vi "Begin.vi"(8 "error in":errorcluster) -> (0 "error out":errorcluster)   [LabVIEW 2020]
doc: "Called before other user functions, this VI is expected to open initial I/O refnums, load in file data, and do all program initialization. Notice that the <B>error out</B> terminal is simply used for data flow. Wiring it to other structures or subVIs ensures that this VI runs first."
uses:
  <vilib>/Rock Robotics/WPI/DriverStation/WPI_DriverStationRobotMode2.ctl
  <vilib>/Rock Robotics/WPI/Joystick/WPI_JoystickDeviceEnum.ctl
  Robot Global Data.vi
  <vilib>/Rock Robotics/WPI/RobotDrive/WPI_RobotDriveOpen2MotorWithExistingMotors.vi
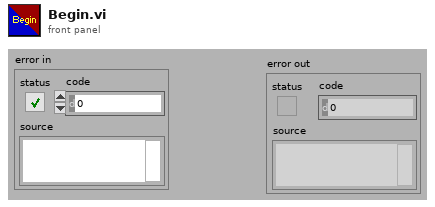
[diagram p1: front panel]
types:
  T1 = typedef "WPI_JoystickDeviceEnum.ctl" = enum16{"USB 0", "USB 1", "USB 2", "USB 3", "USB 4", "USB 5"}
  T2 = typedef "WPI_DriverStationRobotMode2.ctl" = enum16{"Autonomous Disabled", "Autonomous Enabled", "Teleop Disabled", "Teleop Enabled", "Disconnected", "Finish", "Test Disabled", "Test Enabled", "Emergency Stopped"}
  T3 = typedef "WPI_JoystickDevRef.ctl" = cluster{"Device":T1}
  T4 = typedef "WPI_MotorControlDeviceRef.ctl" = cluster{"DeviceStatus":errorcluster, "Type":T5, "PWM":cluster{"PWM Channel":T6, "DeadBand":T7}, "CAN":cluster{"Device Number":u8, "SetOutput VI Ref":variant, "GetOutput VI Ref":variant, "Enable VI Ref":variant, "Disable VI Ref":variant, "Data":variant}, "Invert":bool, "DIO PWM":cluster{"PWM \"Enable\" Channel":T6, "DIOChannel":T8, "PWM Rate":dbl}}
  T5 = typedef "WPI_MotorControlType.ctl" = enum16{"PWM", "CAN", "DIO PWM"}
  T6 = typedef "FPGA_DIOPWMChannel.ctl" = enum8{"PWM 0", "PWM 1", "PWM 2", "PWM 3", "PWM 4", "PWM 5", "PWM 6", "PWM 7", "PWM 8", "PWM 9", "PWM MXP 0", "PWM MXP 1", "PWM MXP 2", "PWM MXP 3", "PWM MXP 4", "PWM MXP 5", "PWM MXP 6", "PWM MXP 7", "PWM MXP 8", "PWM MXP 9", "Invalid"}
  T7 = typedef "WPI_PWMDeadband.ctl" = cluster{"Name":string, "maxPositivePwm":i32, "minPositivePwm":i32, "centerPwm":i32, "maxNegativePwm":i32, "minNegativePwm":i32, "angularRange":u16}
  T8 = typedef "FPGA_DIOChannel.ctl" = enum8{"DIO 0", "DIO 1", "DIO 2", "DIO 3", "DIO 4", "DIO 5", "DIO 6", "DIO 7", "DIO 8", "DIO 9", "DIO MXP 0", "DIO MXP 1", "DIO MXP 2", "DIO MXP 3", "DIO MXP 4", "DIO MXP 5", "DIO MXP 6", "DIO MXP 7", "DIO MXP 8", "DIO MXP 9", "DIO MXP 10", "DIO MXP 11", "DIO MXP 12", "DIO MXP 13", "DIO MXP 14", "DIO MXP 15", "SPI Port CS1", "SPI Port CS2", "SPI Port CS3", "SPI Port MISO", "SPI Port MOSI", "Invalid"}
  T9 = typedef "WPI_RobotDriveDevRef.ctl" = cluster{"DevStatus":errorcluster, "Motors[]":T4[], "Square Inputs":bool, "Max Output":dbl}
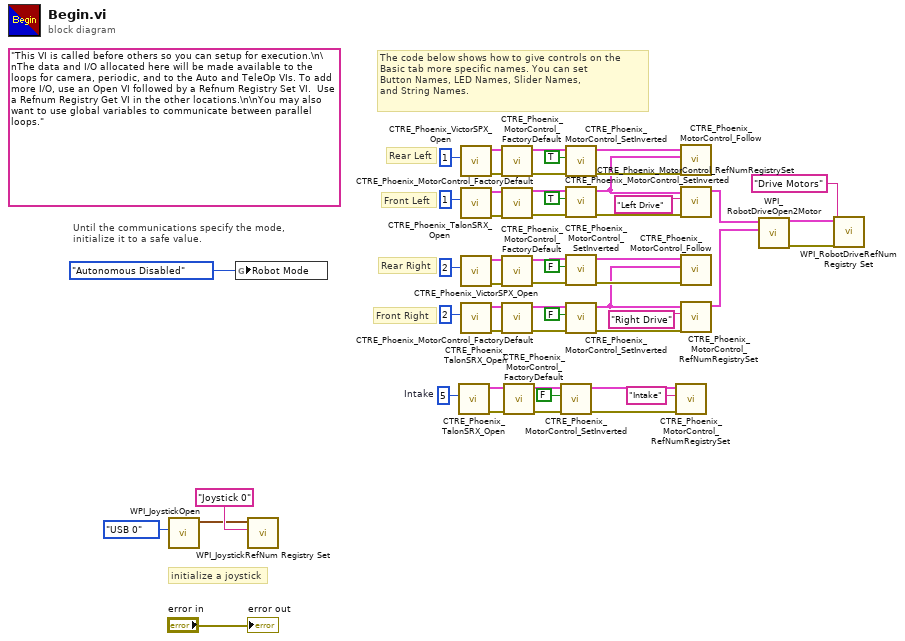
[diagram p0: block diagram]
diagram:
  w3 = u8 5  # Intake
  (unwired) "This VI is called before others so you can setup for execution.\n\nThe data and I/O allocated here will be made available to the loops for camera, periodic, and to the Auto and TeleOp VIs. To add more I/O, use an Open VI followed by a Refnum Registry Set VI.  Use a Refnum Registry Get VI in the other locations.\n\nYou may also want to use global variables to communicate between parallel loops."
  # "Front Right"
  # "Front Left"
  # "Rear Right"
  # "Rear Left"
  # "The code below shows how to give controls on the\nBasic tab more specific names. You can set\nButton Names, LED Names, Slider Names,\nand String Names."
  # "initialize a joystick"
  # "Until the communications specify the mode,\ninitialize it to a safe value."
  n1 = call <vilib>:"WPI_JoystickOpen.vi"("JoystickDevice"=WPI_JoystickDeviceEnum."USB 0") -> ("JoystickDevRef"=w51:T3)  [unwired: 10 in]
  n2 = global write "Robot Global Data.vi" "Robot Mode"(WPI_DriverStationRobotMode2."Autonomous Disabled" ("Robot Mode")) -> ()
  n3 = call <vilib>:"WPI_JoystickRefNum Registry Set.vi"("refnum name"="Joystick 0", "JoystickDevRef"=w51) -> ()  [unwired: 8 in, 2 out]
  n4 = call <vilib>:"CTRE_Phoenix_TalonSRX_Open.vi"("Device Number"=w3) -> ("error out"=w9:errorcluster, "PhoenixMotorControlDevRef"=w8:T4)  [unwired: 9 in]
  n5 = call <vilib>:"CTRE_Phoenix_VictorSPX_Open.vi"("Device Number"=u8 1) -> ("error out"=w37:errorcluster, "PhoenixMotorControlDevRef"=w36:T4)  [unwired: 9 in]
  n6 = call <vilib>:"CTRE_Phoenix_TalonSRX_Open.vi"("Device Number"=u8 1) -> ("error out"=w34:errorcluster, "PhoenixMotorControlDevRef"=w35:T4)  [unwired: 9 in]
  n7 = call <vilib>:"CTRE_Phoenix_VictorSPX_Open.vi"("Device Number"=u8 2) -> ("error out"=w33:errorcluster, "PhoenixMotorControlDevRef"=w32:T4)  [unwired: 9 in]
  n8 = call <vilib>:"CTRE_Phoenix_TalonSRX_Open.vi"("Device Number"=u8 2) -> ("error out"=w31:errorcluster, "PhoenixMotorControlDevRef"=w30:T4)  [unwired: 9 in]
  n9 = call <vilib>:"CTRE_Phoenix_MotorControl_FactoryDefault.vi"("error in"=w37, "PhoenixMotorControlDevRef"=w36) -> ("error out"=w28:errorcluster, "PhoenixMotorControlDevRef"=w27:T4)  [unwired: 8 in]
  n10 = call <vilib>:"CTRE_Phoenix_MotorControl_FactoryDefault.vi"("error in"=w34, "PhoenixMotorControlDevRef"=w35) -> ("error out"=w22:errorcluster, "PhoenixMotorControlDevRef"=w23:T4)  [unwired: 8 in]
  n11 = call <vilib>:"CTRE_Phoenix_MotorControl_FactoryDefault.vi"("error in"=w33, "PhoenixMotorControlDevRef"=w32) -> ("error out"=w18:errorcluster, "PhoenixMotorControlDevRef"=w17:T4)  [unwired: 8 in]
  n12 = call <vilib>:"CTRE_Phoenix_MotorControl_FactoryDefault.vi"("error in"=w31, "PhoenixMotorControlDevRef"=w30) -> ("error out"=w13:errorcluster, "PhoenixMotorControlDevRef"=w12:T4)  [unwired: 8 in]
  n13 = call <vilib>:"CTRE_Phoenix_MotorControl_FactoryDefault.vi"("error in"=w9, "PhoenixMotorControlDevRef"=w8) -> ("error out"=w7:errorcluster, "PhoenixMotorControlDevRef"=w6:T4)  [unwired: 8 in]
  n14 = call <vilib>:"CTRE_Phoenix_MotorControl_SetInverted.vi"("error in (no error)"=w7, "Invert?"=FALSE, "PhoenixMotorControlDevRef"=w6) -> ("error out"=w5:errorcluster, "PhoenixMotorControlDevRef"=w4:T4)  [unwired: 7 in]
  n15 = call <vilib>:"CTRE_Phoenix_MotorControl_SetInverted.vi"("error in (no error)"=w28, "Invert?"=TRUE, "PhoenixMotorControlDevRef"=w27) -> ("error out"=w25:errorcluster, "PhoenixMotorControlDevRef"=w26:T4)  [unwired: 7 in]
  n16 = call <vilib>:"CTRE_Phoenix_MotorControl_SetInverted.vi"("error in (no error)"=w22, "Invert?"=TRUE, "PhoenixMotorControlDevRef"=w23) -> ("error out"=w21:errorcluster, "PhoenixMotorControlDevRef"=w20:T4)  [unwired: 7 in]
  n17 = call <vilib>:"CTRE_Phoenix_MotorControl_SetInverted.vi"("error in (no error)"=w18, "Invert?"=FALSE, "PhoenixMotorControlDevRef"=w17) -> ("error out"=w15:errorcluster, "PhoenixMotorControlDevRef"=w16:T4)  [unwired: 7 in]
  n18 = call <vilib>:"CTRE_Phoenix_MotorControl_SetInverted.vi"("error in (no error)"=w13, "Invert?"=FALSE, "PhoenixMotorControlDevRef"=w12) -> ("error out"=w10:errorcluster, "PhoenixMotorControlDevRef"=w11:T4)  [unwired: 7 in]
  n19 = call <vilib>:"CTRE_Phoenix_MotorControl_RefNumRegistrySet.vi"("error in (no error)"=w5, "refnum name"="Intake", "PhoenixMotorControlDevRef"=w4) -> ()  [unwired: 7 in, 2 out]
  n20 = call <vilib>:"CTRE_Phoenix_MotorControl_Follow.vi"("error in (no error)"=w25, "Master Controller to Follow"=w20, "PhoenixMotorControlDevRef"=w26) -> ()  [unwired: 7 in, 2 out]
  n21 = call <vilib>:"CTRE_Phoenix_MotorControl_RefNumRegistrySet.vi"("error in (no error)"=w21, "refnum name"="Left Drive", "PhoenixMotorControlDevRef"=w20) -> ("PhoenixMotorControlDevRef"=w44:T4)  [unwired: 7 in, 1 out]
  n22 = call <vilib>:"CTRE_Phoenix_MotorControl_Follow.vi"("error in (no error)"=w15, "Master Controller to Follow"=w11, "PhoenixMotorControlDevRef"=w16) -> ()  [unwired: 7 in, 2 out]
  n23 = call <vilib>:"CTRE_Phoenix_MotorControl_RefNumRegistrySet.vi"("error in (no error)"=w10, "refnum name"="Right Drive", "PhoenixMotorControlDevRef"=w11) -> ("PhoenixMotorControlDevRef"=w43:T4)  [unwired: 7 in, 1 out]
  n24 = call-poly <vilib>:"WPI_RobotDriveOpen2Motor.vi"("Right Motor Dev Ref"=w43, "Left Motor Dev Ref"=w44) -> ("error out"=w39:errorcluster, "RobotDriveDevRef"=w40:T9)  [unwired: 8 in]
  n25 = call <vilib>:"WPI_RobotDriveRefNum Registry Set.vi"("error in (no error)"=w39, "refnum name"="Drive Motors", "RobotDriveDevRef"=w40) -> ()  [unwired: 7 in, 2 out]
  "error out" <- "error in"
